vi "Helper Loop.vi"(8 "error in (no error)":errorcluster, 11 "TDMS DAQ in":refnum<class "TDMS DAQ.lvclass">) -> ()   [LabVIEW 2020, in "TDMS DAQ.lvlib" / "TDMS DAQ.lvclass"]
uses:
  TDMS DAQ.lvclass
  C:/Program Files/National Instruments/LabVIEW 2025/vi.lib/ActorFramework/Actor/Actor.lvclass
  Helper Loop State.ctl
  <vilib>/Natan Biesmans/G2CPU GPU and CPU HPC Toolkit/G2CPU Libraries/Async IO/DMA Manager/DMA Manager.lvclass
  Configure TDMS DAQ.ctl
  <vilib>/Platform/TimedLoop/XDataNode/timing_clust.ctl
  <vilib>/Platform/TimedLoop/XDataNode/nitl_modes.ctl
  <vilib>/Platform/TimedLoop/XDataNode/wakeup.ctl
  TDMS DAQ.lvclass/TDMS DAQ.ctl
  Helper Loop Message.ctl
  Helper Loop Type.ctl
  Filled Buffers.ctl
  <vilib>/ActorFramework/Actor/Actor.lvclass/Actor.ctl
  <vilib>/ActorFramework/Message Enqueuer/Message Enqueuer.lvclass/Message Enqueuer.ctl
  DAQ Interface/DAQ Interface Messages/Process Filled Buffer Msg/Process Filled Buffer Msg.lvclass/Process Filled Buffer Msg.ctl
  545e4e43-0907-4128-bf3e-df0c433206dc.vi
  545e4e43-0907-4128-bf3e-df0c433206dc.vi/ba35b323-08e1-4c79-a1ea-61c0f2b0d3b5.vi
  545e4e43-0907-4128-bf3e-df0c433206dc.vi/c1c6ba82-99b7-4273-a704-85eea64f3b4b.vi
  545e4e43-0907-4128-bf3e-df0c433206dc.vi/8aa0c4af-4daa-4014-9a01-595272b02124.vi
  545e4e43-0907-4128-bf3e-df0c433206dc.vi/6d883df8-3b64-4008-8da1-8b1f8b11b48b.vi
  <vilib>/ActorFramework/Message Enqueuer/Init from Existing Queue.vi
  <vilib>/ActorFramework/Message Enqueuer/Enqueue.vi
  545e4e43-0907-4128-bf3e-df0c433206dc.vi/ba35b323-08e1-4c79-a1ea-61c0f2b0d3b5.vi/1a23f98f-393f-4176-8983-7f1ab824c539.vi
  545e4e43-0907-4128-bf3e-df0c433206dc.vi/8aa0c4af-4daa-4014-9a01-595272b02124.vi/c174a7f7-781d-4fed-8bab-bf30bc03dac0.vi
  545e4e43-0907-4128-bf3e-df0c433206dc.vi/6d883df8-3b64-4008-8da1-8b1f8b11b48b.vi/360ddb94-76c6-469a-8529-bee7b421957e.vi
  545e4e43-0907-4128-bf3e-df0c433206dc.vi/6d883df8-3b64-4008-8da1-8b1f8b11b48b.vi/360ddb94-76c6-469a-8529-bee7b421957e.vi/1a23f98f-393f-4176-8983-7f1ab824c539.vi
  <vilib>/Natan Biesmans/G2CPU GPU and CPU HPC Toolkit/G2CPU Libraries/Arrays/1DArray/s16/1D Array s16.lvclass
  C:/Program Files/National Instruments/LabVIEW 2025/vi.lib/Natan Biesmans/G2CPU GPU and CPU HPC Toolkit/G2CPU Libraries/Arrays/Array/Array Prototype.lvclass
  DAQ Interface/DAQ Interface Messages/Process Filled Buffer Msg/Process Filled Buffer Msg.lvclass
  C:/Program Files/National Instruments/LabVIEW 2025/vi.lib/ActorFramework/Message/Message.lvclass
  <vilib>/Natan Biesmans/G2CPU GPU and CPU HPC Toolkit/G2CPU Libraries/Manage Environment/G2CPU Get Backend.vi
  <vilib>/Utility/error.llb/Error Cluster From Error Code.vi
  <vilib>/Natan Biesmans/G2CPU GPU and CPU HPC Toolkit/ArrayFire Driver/VIs/Run as Multi Device.vi
  <vilib>/Natan Biesmans/G2CPU GPU and CPU HPC Toolkit/G2CPU Libraries/Runtime Licensing/G2CPU License Check.vi
  <vilib>/Natan Biesmans/G2CPU GPU and CPU HPC Toolkit/G2CPU Libraries/Manage Environment/Find AF DLL.vi
  <vilib>/Natan Biesmans/G2CPU GPU and CPU HPC Toolkit/G2CPU Libraries/Arrays/Array/G2CPU Set Array Pointer.vi
  <resource>/Natan Biesmans/G2CPU GPU and CPU HPC Toolkit/Garbage Collector/G2CPU DMAGarbageCollectorFGV.vi
  <vilib>/ActorFramework/Message Priority Queue/Priority Enqueue.vi
  <vilib>/platform/TimedLoop/XDataNode/XDataNode.xnode
  <vilib>/Natan Biesmans/G2CPU GPU and CPU HPC Toolkit/G2CPU Libraries/Arrays/Array/Array Prototype.lvclass
  <vilib>/ActorFramework/Message Enqueuer/Message Enqueuer.lvclass
  <vilib>/Platform/TimedLoop/XDataNode/XDNodeRunTimeDep.lvlib
  DAQ Interface/DAQ Interface/DAQ Interface.lvclass
  <vilib>/ActorFramework/Actor/Actor.lvclass
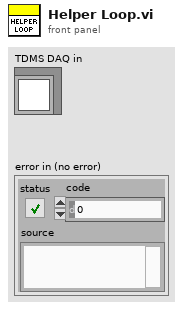
[diagram p1: front panel]
types:
  T1 = typedef "TDMS DAQ.lvlib/TDMS DAQ.lvclass/Helper Loop State.ctl" = cluster{"Stop":bool, "DMA Buffer Queue":refnum<queue>, "DMA Manager":refnum<class "DMA Manager.lvclass">, "Config":T2}
  T2 = typedef "TDMS DAQ.lvlib/TDMS DAQ.lvclass/Configure TDMS DAQ.ctl" = cluster{"Path":path, "Thread Count":i32, "Batch Size":i32}
  T3 = typedef "TDMS DAQ.lvlib/TDMS DAQ.lvclass/Helper Loop Message.ctl" = cluster{"Type":T4, "Payload":variant}
  T4 = typedef "TDMS DAQ.lvlib/TDMS DAQ.lvclass/Helper Loop Type.ctl" = enum16{"Configure", "Start", "Do", "Stop", "Clean", "Close"}
  T5 = typedef "DAQ Interface.lvlib/DAQ Interface.lvclass/Filled Buffers.ctl" = cluster{"DMA Manager":refnum<class "DMA Manager.lvclass">, "DMA Memory":refnum<data-value>, "Gain":dbl, "dt":dbl, "f0":dbl}
  T6 = enum16{"open", "open or create", "create or replace", "create", "open (read-only)"}
  T7 = typedef "XDNodeRunTimeDep.lvlib/timing_clust.ctl" = cluster{"Expected End [f-1]":u64, "Actual End [f-1]":u64, "Finished Late? [f-1]":bool, "Expected End [i-1]":u64, "Actual End [i-1]":u64, "Finished Late? [i-1]":bool, "Expected Start [i]":u64, "Actual Start [i]":u64, "Expected Start [f]":u64, "Actual Start [f]":u64, "Source Name":string, "Structure Name":string, "Period":i64, "Deadline":i64, "Offset":i64, "Start":i64, "Priority":i32, "Timeout":i32, "Mode":T8, "Wakeup Reason":T9, "Error":errorcluster, "Source Type":string, "Secondary Source Type":string, "Global End Time":u64, "Global Start Time":u64, "Frame Duration":u64, "Iteration Duration":u64, "Assigned CPU":i32, "I/O Scan Engine Mode":u32}
  T8 = typedef "XDNodeRunTimeDep.lvlib/nitl_modes.ctl" = enum32{"No Change", "Process missed periods, maintain original phase", "Discard missed periods, maintain original phase", "Process missed periods, ignore original phase", "Discard missed periods, ignore original phase"}
  T9 = typedef "XDNodeRunTimeDep.lvlib/wakeup.ctl" = enum32{"Normal", "Aborted", "Asynchronous wakeup", "Timing source error", "Timed loop error", "Timeout"}
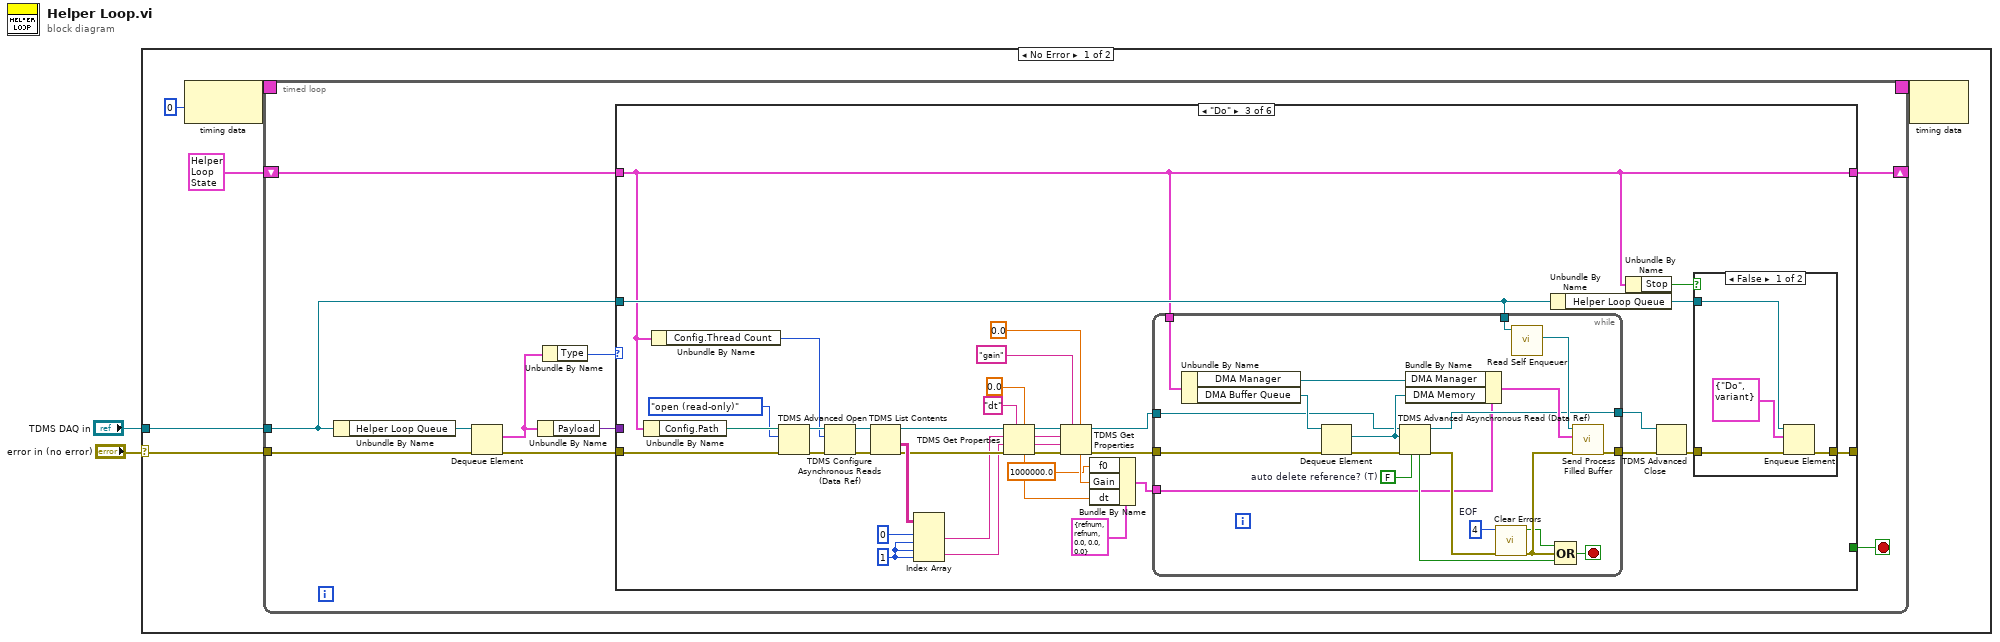
[diagram p0: block diagram]
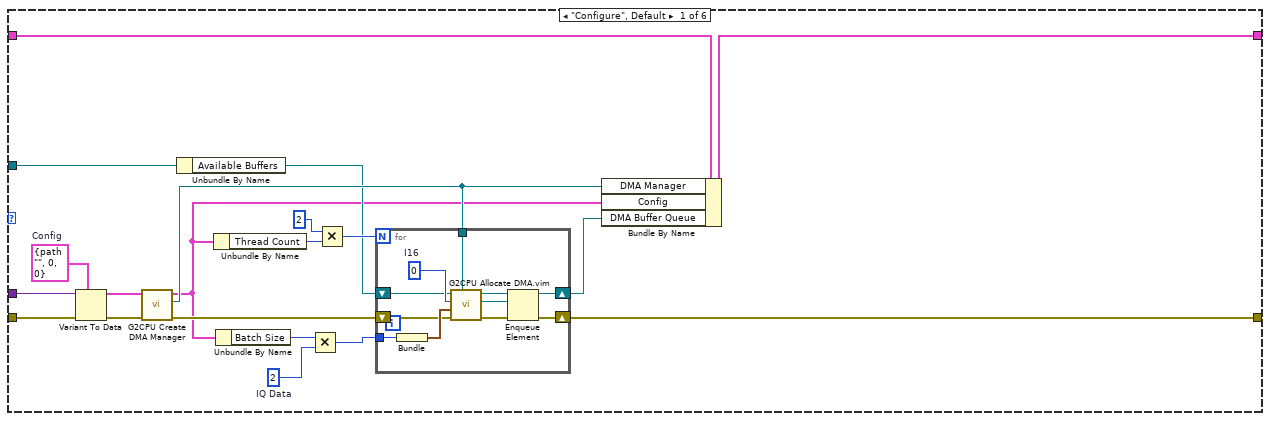
[diagram p2: hidden frame]
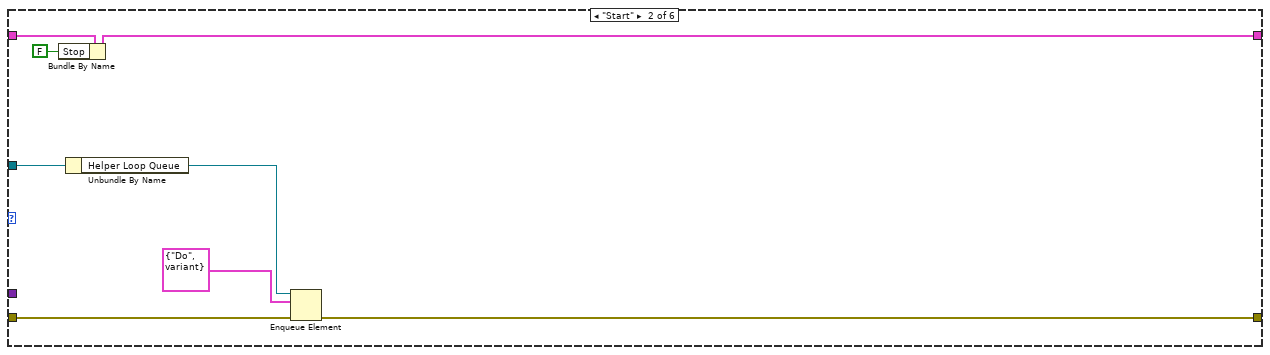
[diagram p3: hidden frame]
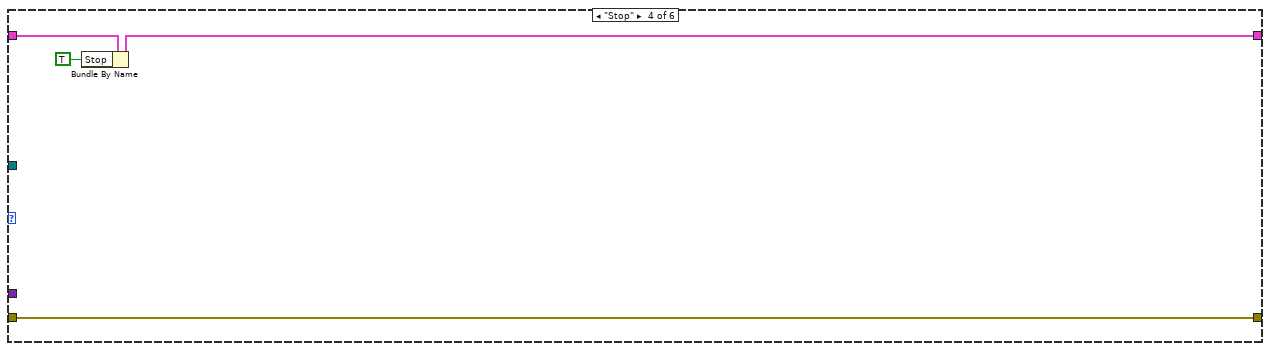
[diagram p5: hidden frame]
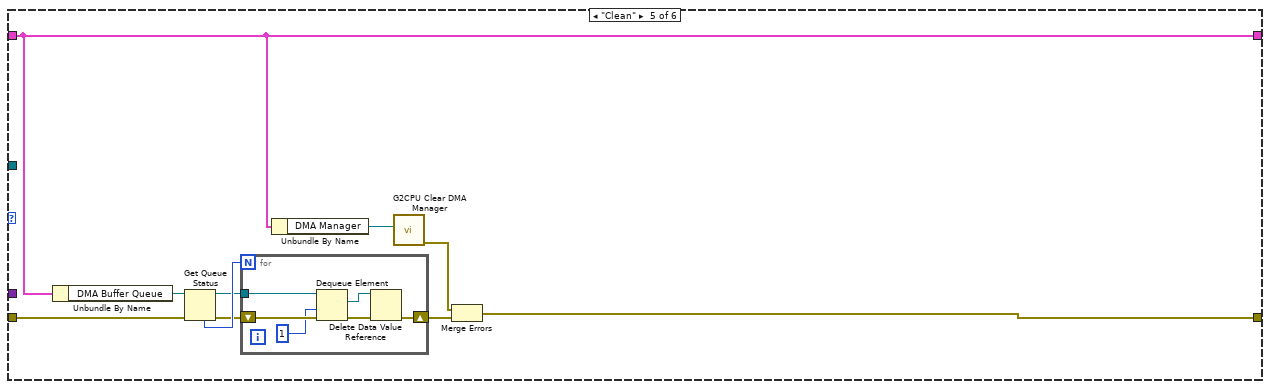
[diagram p6: hidden frame]
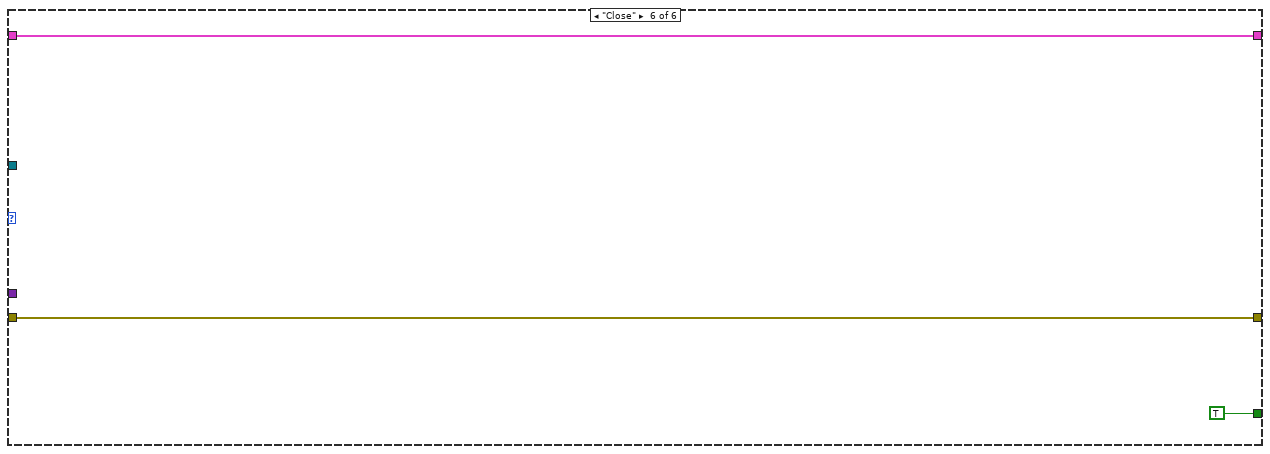
[diagram p7: hidden frame]
diagram:
  n1 = case shown="No Error" "error in (no error)" {
    selector: "error in (no error)" -> [w7 _]
    tunnel: "TDMS DAQ in" -> [w8 _]
    frame No Error {
      n2 = node-c288(i64 0 ("Period")) -> (w6:T7)
      n3 = timed-loop {
        tunnel: w8 -> [w10]
        tunnel: w7 -> [w17]
        timing: w6 -> [_]
        timing-out: [_] -> w5
        shift-right: [w12] -> _
        shift-left: T1 {"Stop"=FALSE, "DMA Buffer Queue"=refnum, "DMA Manager"=refnum, "Config"={"Path"=path "", "Thread Count"=0, "Batch Size"=0}} ("output cluster 2") -> [w11]
        stop <- w9 stop-if-true
        n4 = Unbundle By Name(w10) -> ("Helper Loop Queue"=w18:refnum<queue>)
        n5 = Dequeue Element(queue=w18, error in (no error)=w17) -> (element=w14:T3, error out=w15:errorcluster)  [unwired: 1 in, 2 out]
        n6 = Unbundle By Name(w14) -> ("Payload"=w13:variant)
        n7 = Unbundle By Name(w14) -> ("Type"=w16:T4)
        n8 = case shown="\"Do\"" w16 {
          tunnel: [_ _ _ _ _ TRUE] -> w9
          tunnel: w15 -> [w37 w50 w86 w122 w131 w139]
          tunnel: w13 -> [w36 _ _ _ _ _]
          tunnel: [w33 w49 w93 w122 w126 w139] -> _
          tunnel: [w28 w54 w84 w119 w129 w140] -> w12
          tunnel: w11 -> [w29 w55 w84 w120 w129 w140]
          tunnel: w10 -> [w24 w52 w90 _ _ _]
          frame "Configure", Default {
            w19 = 2  # IQ Data
            w35 = T2 {"Path"=path "", "Thread Count"=0, "Batch Size"=0}  # Config
            n9 = Variant To Data(error in=w37, type=w35, Variant=w36) -> (data=w21:T2, error out=w26:errorcluster)
            n10 = call <vilib>:"G2CPU Create DMA Manager.vi"("error in (no error)"=w26) -> ("error out"=w22:errorcluster, "DMA Manager"=w25:refnum<class "DMA Manager.lvclass">)  [unwired: 9 in]
            n11 = Unbundle By Name(w24) -> ("Available Buffers"=w23:refnum<queue>)
            n12 = Unbundle By Name(w21) -> ("Thread Count"=w32:i32)
            n13 = Unbundle By Name(w21) -> ("Batch Size"=w34:i32)
            n14 = Multiply(x=w34, y=w19) -> (x*y=w20:i32)
            n15 = Multiply(x=2, y=w32) -> (x*y=w31:i32)
            n16 = for {
              N: w31 -> [_]
              tunnel: w25 -> [w47]
              tunnel: w20 -> [w44]
              shift-right: [w41] -> w33
              shift-left: w22 -> [w43]
              shift-right: [w40] -> w27
              shift-left: w23 -> [w39]
              w46 = i16 0  # I16
              n17 = Bundle(w44) -> (w45:cluster{i32})  [unwired: 1 in]
              n18 = call "G2CPU Allocate DMA.vim"("DMA Manager"=w47, "error in (no error)"=w43, "Size"=w45, "Datatype"=w46) -> ("error out"=w42:errorcluster, "DMA Memory"=w38:refnum<data-value>)  [unwired: 6 in]
              n19 = Enqueue Element(queue=w39, element=w38, error in (no error)=w42) -> (queue out=w40:refnum<queue>, error out=w41:errorcluster)  [unwired: 1 in, 1 out]
            }
            n20 = Bundle By Name(cluster=w29, "DMA Manager"=w25, "Config"=w21, "DMA Buffer Queue"=w27) -> (w28:T1)
          }
          frame "Start" {
            n21 = Bundle By Name(cluster=w55, "Stop"=FALSE) -> (w54:T1)
            n22 = Unbundle By Name(w52) -> ("Helper Loop Queue"=w51:refnum<queue>)
            n23 = Enqueue Element(queue=w51, element=T3 {"Type"=enum."Do", "Payload"=variant}, error in (no error)=w50) -> (error out=w49:errorcluster)  [unwired: 1 in, 2 out]
          }
          frame "Do" {
            w79 = 1 ("disabled index (col)")
            n24 = Unbundle By Name(w84) -> ("Config.Path"=w87:path)
            n25 = Unbundle By Name(w84) -> ("Config.Thread Count"=w81:i32)
            n26 = TDMS Advanced Open(8:w86, 10:T6."open (read-only)" ("operation (0:open)"), 11:w87) -> (0:w82:errorcluster, 3:w83:refnum<k34>)  [unwired: 2 in, 1 out]
            n27 = TDMS Configure Asynchronous Reads (Data Ref)(8:w82, 10:w81, 11:w83) -> (0:w67:errorcluster, 3:w68:refnum<k34>)  [unwired: 2 in]
            n28 = TDMS List Contents(4:w67, 7:w68) -> (0:w65:errorcluster, 1:w77:string[][], 3:w66:refnum<k34>)  [unwired: 1 in, 1 out]
            n29 = Index Array(array=w77, index (row) #1=0 ("index (row)"), index (col) #1=w79, index (row) #2=w79, index (col) #2=w79) -> (element #1=w62:string, element #2=w61:string)
            n30 = TDMS Get Properties(5:0.0, 7:"dt" ("property name"), 8:w65, 9:w61, 10:w62, 11:w66) -> (0:w72:errorcluster, 1:w74:string, 2:w73:string, 3:w71:refnum<k34>, 4:w58:dbl)  [unwired: 1 out]
            n31 = TDMS Get Properties(5:0.0, 7:"gain" ("property name"), 8:w72, 9:w74, 10:w73, 11:w71) -> (0:w64:errorcluster, 3:w63:refnum<k34>, 4:w59:dbl)  [unwired: 3 out]
            n32 = Bundle By Name(cluster=T5 {"DMA Manager"=refnum, "DMA Memory"=refnum, "Gain"=0.0, "dt"=0.0, "f0"=0.0} ("element"), "f0"=1000000.0, "Gain"=w59, "dt"=w58) -> (w57:T5)
            n33 = while {
              tunnel: w64 -> [w114]
              tunnel: w84 -> [w118]
              tunnel: [w107] -> w89
              tunnel: w90 -> [w106]
              tunnel: w63 -> [w101]
              tunnel: [w100] -> w80
              tunnel: w57 -> [w99]
              stop <- w117 stop-if-true
              w103 = 4  # EOF
              w115 = FALSE  # auto delete reference? (T)
              n34 = Unbundle By Name(w118) -> ("DMA Manager"=w110:refnum<class "DMA Manager.lvclass">, "DMA Buffer Queue"=w112:refnum<queue>)
              n35 = Dequeue Element(queue=w112, error in (no error)=w114) -> (element=w111:refnum<data-value>, error out=w113:errorcluster)  [unwired: 1 in, 2 out]
              n36 = TDMS Advanced Asynchronous Read (Data Ref)(6:w115, 8:w113, 10:w111, 11:w101) -> (0:w108:errorcluster, 3:w100:refnum<k34>, 4:w116:bool)
              n37 = Bundle By Name(cluster=w99, "DMA Manager"=w110, "DMA Memory"=w111) -> (w109:T5)
              n38 = call <vilib>:"Clear Errors.vi"("error in (no error)"=w108, "specific error code to clear (0: all)"=w103) -> ("error out"=w104:errorcluster, "specific error cleared?"=w102:bool)  [unwired: 4 in]
              n39 = call <vilib>:"Read Self Enqueuer.vi"("Actor"=w106) -> ("Self Enqueuer"=w105:refnum<class "Message Enqueuer.lvclass">)  [unwired: 10 in]
              n40 = Compound Arithmetic op=OR(w102, w104, w116) -> (w117:bool)
              n41 = call "Send Process Filled Buffer.vi"("error in (no error)"=w104, "Filled Buffers"=w109, "Message Enqueuer"=w105) -> ("error out"=w107:errorcluster)  [unwired: 7 in, 1 out]
            }
            n42 = Unbundle By Name(w90) -> ("Helper Loop Queue"=w92:refnum<queue>)
            n43 = Unbundle By Name(w84) -> ("Stop"=w91:bool)
            n44 = TDMS Advanced Close(8:w89, 11:w80) -> (0:w88:errorcluster)  [unwired: 2 in, 1 out]
            n45 = case shown="False" w91 {
              tunnel: w88 -> [w96 w98]
              tunnel: [w95 w98] -> w93
              tunnel: w92 -> [w94 _]
              frame False {
                n46 = Enqueue Element(queue=w94, element=T3 {"Type"=enum."Do", "Payload"=variant}, error in (no error)=w96) -> (error out=w95:errorcluster)  [unwired: 1 in, 2 out]
              }
              frame True {
              }
            }
          }
          frame "Stop" {
            n47 = Bundle By Name(cluster=w120, "Stop"=TRUE) -> (w119:T1)
          }
          frame "Clean" {
            n48 = Unbundle By Name(w129) -> ("DMA Buffer Queue"=w132:refnum<queue>)
            n49 = Get Queue Status(queue=w132, error in (no error)=w131) -> (queue out=w123:refnum<queue>, error out=w124:errorcluster, # elements in queue=w130:i32)  [unwired: 1 in, 5 out]
            n50 = for {
              N: w130 -> [_]
              shift-right: [w138] -> w125
              shift-left: w124 -> [w136]
              tunnel: w123 -> [w137]
              n51 = Dequeue Element(queue=w137, timeout in ms (-1)=1, error in (no error)=w136) -> (element=w135:refnum<data-value>, error out=w134:errorcluster)  [unwired: 2 out]
              n52 = Delete Data Value Reference(data value reference=w135, error in=w134) -> (error out=w138:errorcluster)  [unwired: 1 out]
            }
            n53 = Unbundle By Name(w129) -> ("DMA Manager"=w128:refnum<class "DMA Manager.lvclass">)
            n54 = call <vilib>:"G2CPU Clear DMA Manager.vi"("DMA Manager"=w128) -> ("error out"=w127:errorcluster)  [unwired: 10 in]
            n55 = Merge Errors(w127, w125) -> (w126:errorcluster)
          }
          frame "Close" {
          }
        }
      }
      n56 = node-c288(w5) -> ()  [unwired: 1 out]
    }
    frame Error {
    }
  }
